vi "View Update Duration.vi"(8 "error in (no error)":errorcluster, 10 "Duration":dbl, 11 "Chef View in":refnum<class "Chef View.lvclass">) -> (0 "error out":errorcluster, 3 "Chef View out":refnum<class "Chef View.lvclass">)   [LabVIEW 2024, in "Chef View.lvlib" / "Chef View.lvclass"]
uses:
  Chef View.lvclass
  Chef View.lvclass/Chef View.ctl
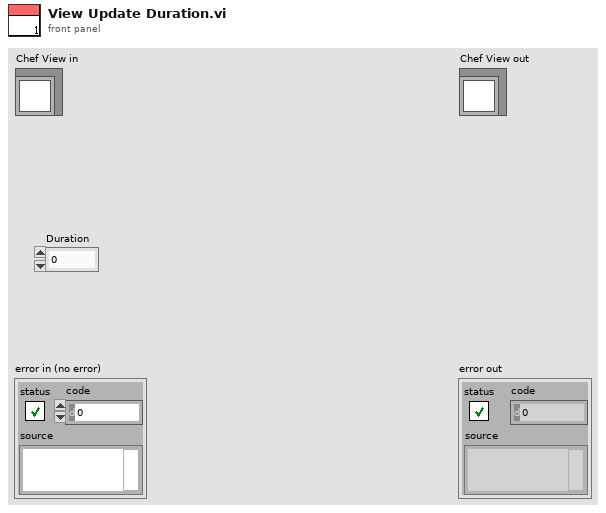
[diagram p1: front panel]
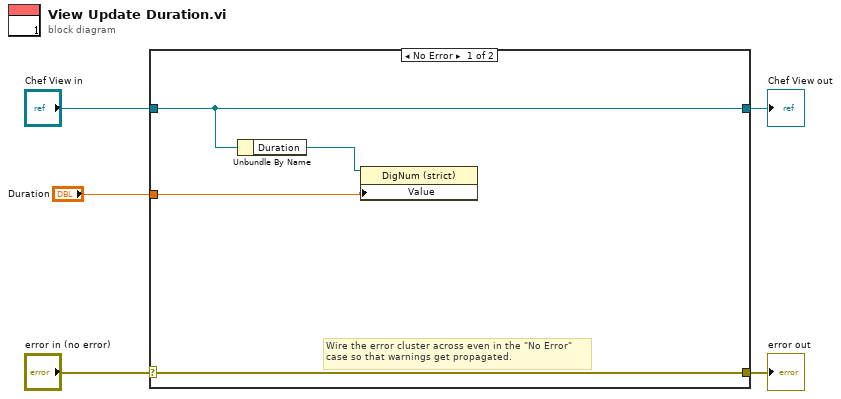
[diagram p0: block diagram]
diagram:
  n1 = case shown="No Error" "error in (no error)" {
    selector: "error in (no error)" -> [w9 w11]
    tunnel: [w9 w11] -> w4
    tunnel: [w8 w10] -> w2
    tunnel: "Chef View in" -> [w8 w10]
    tunnel: "Duration" -> [w6 _]
    frame No Error {
      # "Wire the error cluster across even in the \"No Error\"\ncase so that warnings get propagated."
      n2 = Unbundle By Name(w8) -> ("Duration"=w7:refnum<vi>)
      n3 = property class="DigNum (strict)"(reference=w7, "Value"=w6) -> ()  [unwired: 1 in, 2 out]
    }
    frame Error {
    }
  }
  "error out" <- w4
  "Chef View out" <- w2
